vi "PH_Cam_BaseClass.set GUI Refs.vi"(0 "VI in":refnum<vi>, 2 "Class":string, 3 "GUI Refs to set":T2, 5 "error in (no error)":errorcluster) -> (14 "VI out":refnum<vi>, 19 "error out":errorcluster)   [LabVIEW 2014, in "PH_Cam_BaseClass.lvlib"]
uses:
  PH_Cam_BaseClass.lvlib
  PH_Cam_BaseClass.GUI Refs.ctl
  PH_PSDBWriter/PH_PSDBWriter.lvlib
  PH_StatusHandler/PH_StatusHandler.lvlib
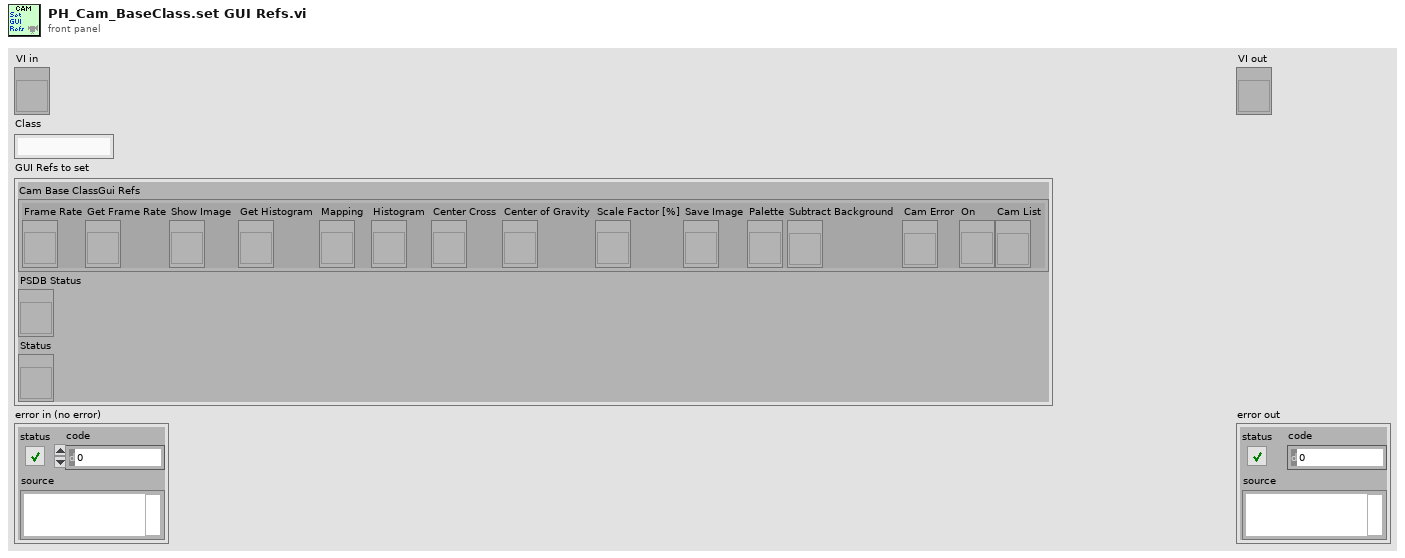
[diagram p1: front panel]
types:
  T1 = typedef "PH_Cam_BaseClass.lvlib/PH_Cam_BaseClass.GUI Refs.ctl" = cluster{"Frame Rate":refnum<vi>, "Get Frame Rate":refnum<vi>, "Show Image":refnum<vi>, "Get Histogram":refnum<vi>, "Mapping":refnum<vi>, "Histogram":refnum<vi>, "Center Cross":refnum<vi>, "Center of Gravity":refnum<vi>, "Scale Factor [%]":refnum<vi>, "Save Image":refnum<vi>, "Palette":refnum<vi>, "Subtract Background":refnum<vi>, "Cam Error":refnum<vi>, "On":refnum<vi>, "Cam List":refnum<vi>}
  T2 = cluster{"Cam Base ClassGui Refs":T1, "PSDB Status":refnum<vi>, "Status":refnum<vi>}
  T3 = typedef "PH_Cam_BaseClass.lvlib/PH_Cam_BaseClass.i attribute.ctl" = cluster{"Gui Refs":T1, "Cam":cluster{"Source Notifier":refnum<notifier>, "Error":errorcluster, "Camera ID":string}, "Images":cluster{"Cam":T4, "Operation":T4, "PSDB":T4}, "Window Image":cluster{"Indicate Image":bool, "Window No.":i32, "Scale Facor":dbl, "Center Cross":bool, "Subtract Backgr":bool, "CoG":bool, "Color Palette":cluster{"Red":u8, "Green":u8, "Blue":u8}[], "Image On":bool}, "Default Prdc Int":i32, "Performance":cluster{"on":bool, "Timestamp Last Frame":i32}, "Histogram":cluster{"on":bool, "Mapping":bool}, "Save Image":cluster{"Save":bool, "File refnum":refnum<file>}, "Setting Service ID":i32, "Screen":cluster{"x-resolution":i16, "y-resolution":i16}, "On":bool, "Constructor finished":bool, "configured":bool}
  T4 = typedef "IMAQ Image.ctl" = refnum<image>
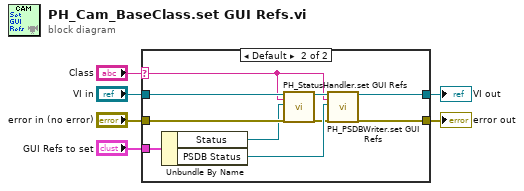
[diagram p0: block diagram]
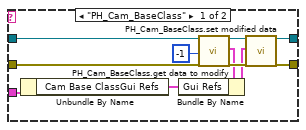
[diagram p2: hidden frame]
diagram:
  n1 = case shown="Default" "Class" {
    selector: "Class" -> [_ w19]
    tunnel: [w9 w27] -> w6
    tunnel: "error in (no error)" -> [w10 w26]
    tunnel: [w11 w25] -> w5
    tunnel: "VI in" -> [w12 w21]
    tunnel: "GUI Refs to set" -> [w8 w24]
    frame "PH_Cam_BaseClass" {
      n2 = Unbundle By Name(w8) -> ("Cam Base ClassGui Refs"=w7:T1)
      n3 = call "PH_Cam_BaseClass.get data to modify.vi"("i ref in"=w12, "ms timeout (10000)"=-1, "error in (no error)"=w10) -> ("i ref out"=w17:refnum<vi>, "i attribute"=w14:T3, "error out"=w16:errorcluster)  [unwired: 13 in, 1 out]
      n4 = Bundle By Name(cluster=w14, "Gui Refs"=w7) -> (w13:T3)
      n5 = call "PH_Cam_BaseClass.set modified data.vi"("i ref in"=w17, "i attribute"=w13, "error in (no error)"=w16) -> ("i ref out"=w11:refnum<vi>, "error out"=w9:errorcluster)  [unwired: 15 in]
    }
    frame Default {
      n6 = Unbundle By Name(w24) -> ("Status"=w18:refnum<vi>, "PSDB Status"=w23:refnum<vi>)
      n7 = call "PH_StatusHandler.set GUI Refs.vi"("i ref in"=w21, "Class"=w19, "GUI Ref"=w18, "error in (no error)"=w26) -> ("i ref out"=w20:refnum<vi>, "error out"=w22:errorcluster)  [unwired: 14 in]
      n8 = call "PH_PSDBWriter.set GUI Refs.vi"("i ref in"=w20, "Class"=w19, "Ref PSDB Status"=w23, "error in"=w22) -> ("i ref out"=w25:refnum<vi>, "error out"=w27:errorcluster)  [unwired: 14 in]
    }
  }
  "error out" <- w6
  "VI out" <- w5
